vi "Read Loop Async.vi"(11 "Chat Client in":refnum<class "Chat Client.lvclass">) -> ()   [LabVIEW 2020, in "Chat Client.lvclass"]
uses:
  Chat Client.lvclass
  Chat Client.lvclass/Chat Client.ctl
  Stream-TCP/TCP Client/TCP Client.lvclass
  lv-stream/stream/Stream/Stream.lvclass
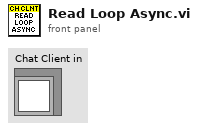
[diagram p1: front panel]
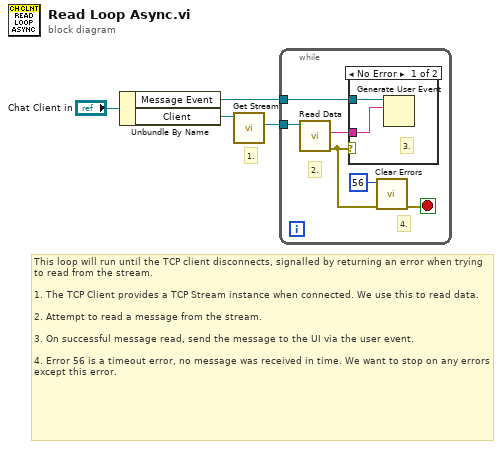
[diagram p0: block diagram]
diagram:
  # "This loop will run until the TCP client disconnects, signalled by returning an error when trying to read from the stream.\n\n1. The TCP Client provides a TCP Stream instance when connected. We use this to read data.\n\n2. Attempt to read a message from the stream.\n\n3. On successful message read, send the message to the UI via the user event.\n\n4. Error 56 is a timeout error, no message was received in time. We want to stop on any errors except this error."
  # "1."
  n1 = Unbundle By Name("Chat Client in") -> ("Message Event"=w1:refnum<user-event>, "Client"=w3:refnum<class "TCP Client.lvclass">)
  n2 = call-dynamic "Get Stream.vi"("TCP Client in"=w3) -> ("Stream"=w2:refnum<class "Stream.lvclass">)  [unwired: 8 in, 2 out]
  n3 = while {
    tunnel: w2 -> [w10]
    tunnel: w1 -> [w7]
    stop <- w6 stop-if-true
    # "4."
    # "2."
    n4 = call-dynamic "Read Data.vi"("Stream in"=w10) -> ("error out"=w9:errorcluster, "Data"=w8:string)  [unwired: 8 in, 1 out]
    n5 = case shown="No Error" w9 {
      tunnel: w8 -> [w11 _]
      tunnel: w7 -> [w12 _]
      frame No Error {
        # "3."
        n6 = Generate User Event(user event=w12, event data cluster=w11) -> ()  [unwired: 2 in, 2 out]
      }
      frame Error {
      }
    }
    n7 = call <vilib>:"Clear Errors.vi"("error in (no error)"=w9, "specific error code to clear (0: all)"=56) -> ("error out"=w6:errorcluster)  [unwired: 4 in, 1 out]
  }
